vi "CoerceOutOfBound.vi"(11 "Rectangle":T1) -> (3 "Coerced Rectangle":T1)   [LabVIEW 2025, in "Picture2D.lvlib"]
uses:
  Picture2D/Picture2D.lvlib
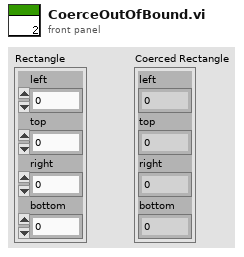
[diagram p1: front panel]
types:
  T1 = cluster{"left":i16, "top":i16, "right":i16, "bottom":i16}
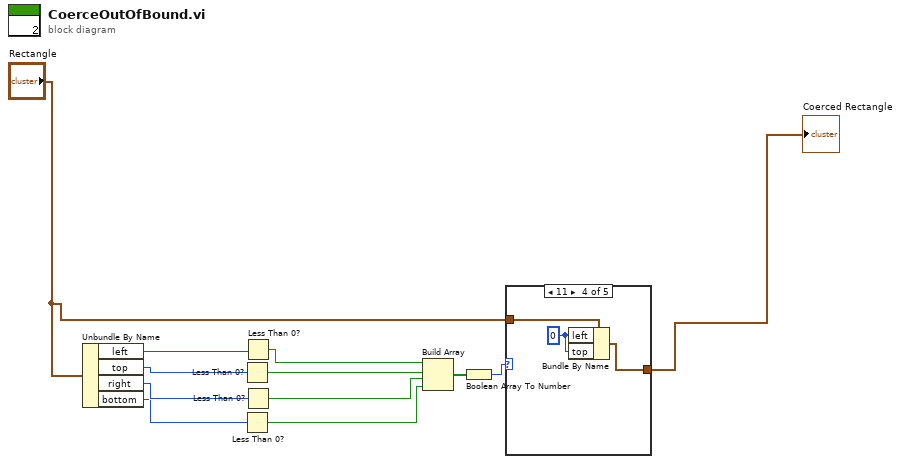
[diagram p0: block diagram]
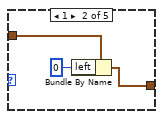
[diagram p3: hidden frame]
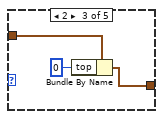
[diagram p4: hidden frame]
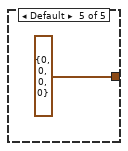
[diagram p5: hidden frame]
diagram:
  n1 = Unbundle By Name("Rectangle") -> ("left"=w12:i16, "top"=w8:i16, "right"=w7:i16, "bottom"=w6:i16)
  n2 = Less Than 0?(x=w8) -> (x < 0?=w5:bool)
  n3 = Less Than 0?(x=w6) -> (x < 0?=w3:bool)
  n4 = Less Than 0?(x=w12) -> (x < 0?=w9:bool)
  n5 = Less Than 0?(x=w7) -> (x < 0?=w4:bool)
  n6 = Build Array(w9, w5, w4, w3) -> (w11:bool[])
  n7 = Boolean Array To Number(Boolean array=w11) -> (number=w10:u32)
  n8 = case shown="11" w10 {
    tunnel: [w13 w14 w17 w21 T1 {"left"=0, "top"=0, "right"=0, "bottom"=0} ("Rectangle")] -> w2
    tunnel: "Rectangle" -> [w13 w16 w19 w22 _]
    frame 0 {
    }
    frame 1 {
      n9 = Bundle By Name(cluster=w16, "left"=i16 0) -> (w14:T1)
    }
    frame 2 {
      n10 = Bundle By Name(cluster=w19, "top"=i16 0 ("left")) -> (w17:T1)
    }
    frame 3 {
      w20 = i16 0 ("left")
      n11 = Bundle By Name(cluster=w22, "left"=w20, "top"=w20) -> (w21:T1)
    }
    frame Default {
    }
  }
  "Coerced Rectangle" <- w2
